vi "GetCurrent.vi"(4 "error in":errorcluster, 5 "connection ID":refnum<k5>) -> (0 "Current":string, 1 "error out":errorcluster, 2 "connection ID out":refnum<k5>, 3 "Answer":bool)   [LabVIEW 2013]
panel:
  out "читаю hex":string
  out "читаю текст":string
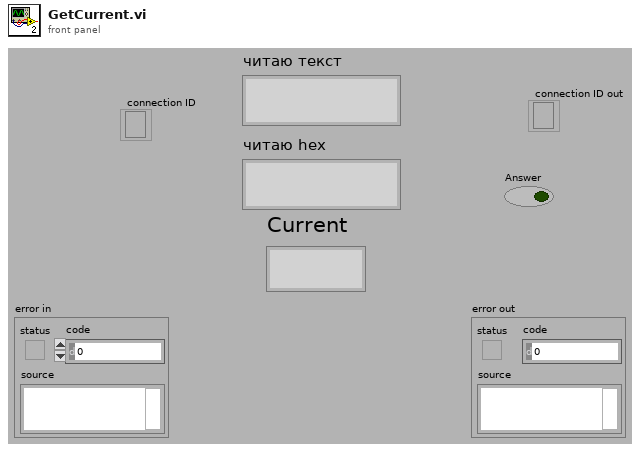
[diagram p1: front panel]
types:
  T1 = enum16{"Standard", "Buffered", "CRLF", "Immediate"}
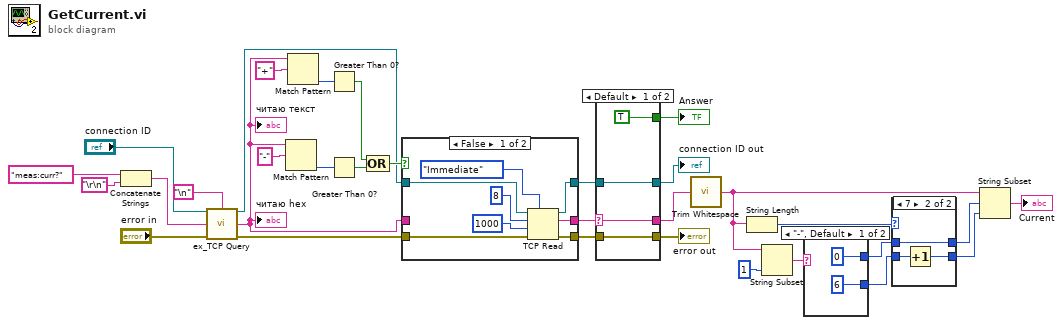
[diagram p0: block diagram]
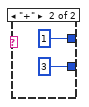
[diagram p3: hidden frame]
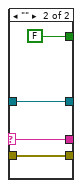
[diagram p5: hidden frame]
diagram:
  n1 = Concatenate Strings("meas:curr?" ("data in"), "\r\n") -> (w7:string)
  n2 = call "ex_TCP Query.vi"("TCP Network Connection in"="connection ID", "Termination character"="\n", "Query string"=w7, "error in (no error)"="error in") -> ("TCP Network Connection out"=w3:refnum<k5>, "Message data out"=w1:string, "error out"=w2:errorcluster)  [unwired: 8 in, 1 out]
  "читаю hex" <- w1
  "читаю текст" <- w1
  n3 = Match Pattern(string=w1, regular expression="-") -> (offset past match=w21:i32)  [unwired: 1 in, 3 out]
  n4 = Match Pattern(string=w1, regular expression="+") -> (offset past match=w30:i32)  [unwired: 1 in, 3 out]
  n5 = Greater Than 0?(x=w30) -> (x > 0?=w20:bool)
  n6 = Greater Than 0?(x=w21) -> (x > 0?=w19:bool)
  n7 = Compound Arithmetic op=OR(w20, w19) -> (w18:bool)
  n8 = case shown="False" w18 {
    tunnel: w1 -> [_ w43]
    tunnel: [w33 w43] -> w25
    tunnel: w3 -> [w37 w42]
    tunnel: [w36 w42] -> w24
    tunnel: w2 -> [w35 w41]
    tunnel: [w34 w41] -> w23
    frame False {
      n9 = TCP Read(connection ID=w37, bytes to read=8, error in (no error)=w35, 7:T1."Immediate" ("mode (standard)"), 9:1000 ("timeout ms (25000)")) -> (connection ID out=w36:refnum<k5>, data out=w33:string, error out=w34:errorcluster)
    }
    frame True {
    }
  }
  n10 = case shown="Default" w25 {
    selector: w25 -> [w47 w51]
    tunnel: [w47 w51] -> w16
    tunnel: [TRUE FALSE] -> w26
    tunnel: w23 -> [w45 w49]
    tunnel: [w45 w49] -> w28
    tunnel: w24 -> [w44 w48]
    tunnel: [w44 w48] -> w29
    frame Default {
    }
    frame "" {
    }
  }
  "Answer" <- w26
  "connection ID out" <- w29
  "error out" <- w28
  n11 = call <vilib>:"Trim Whitespace.vi"("string"=w16) -> ("trimmed string"=w13:string)  [unwired: 1 in]
  n12 = String Length(string=w13) -> (length=w12:i32)
  n13 = String Subset(string=w13, length (rest)=1 ("length (rest)")) -> (substring=w15:string)  [unwired: 1 in]
  n14 = case shown="\"-\", Default" w15 {
    tunnel: [0 ("length (rest)") 1 ("length (rest)")] -> w9
    tunnel: [6 ("length (rest)") 3 ("length (rest)")] -> w11
    frame "-", Default {
    }
    frame "+" {
    }
  }
  n15 = case shown="7" w12 {
    tunnel: w11 -> [w57 w60]
    tunnel: [w57 w59] -> w10
    tunnel: w9 -> [w56 w58]
    tunnel: [w56 w58] -> w8
    frame 6, Default {
    }
    frame 7 {
      n16 = Increment(x=w60) -> (x+1=w59:i32)
    }
  }
  n17 = String Subset(string=w13, offset (0)=w8, length (rest)=w10) -> (substring=→"Current":string)
